vi "Convert Time Stamp to String.vi"(10 "time stamp":timestamp format="%<%Y-%m-%dT%H:%M:%S%8u\nTime zone offset %z>T") -> (3 "date/time string":string)   [LabVIEW 2019, in "infolib.lvlib"]
uses:
  infolib.lvlib
  <vilib>/Utility/miscctls.llb/LVDateTimeRec.ctl
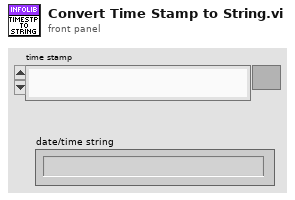
[diagram p1: front panel]
types:
  T1 = typedef "LVDateTimeRec.ctl" = cluster{"fractional second":dbl, "second":i32, "minute":i32, "hour":i32, "day of month":i32, "month":i32, "year":i32, "day of week":i32, "day of year":i32, "DST":i32}
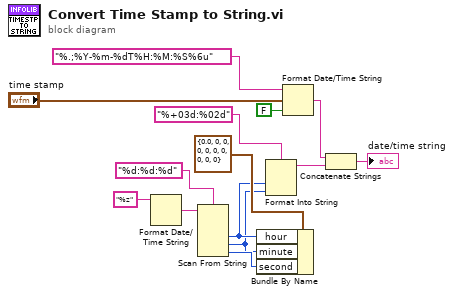
[diagram p0: block diagram]
diagram:
  n1 = Format Date/Time String(time format string (%c)="%z") -> (date/time string=w11:string)  [unwired: 2 in]
  n2 = Scan From String(format string="%d:%d:%d", input string=w11) -> (output 1=w5:i32, output 2=w4:i32, output 3=w8:i32)  [unwired: 5 in, 3 out]
  n3 = Bundle By Name(cluster=T1 {"fractional second"=0.0, "second"=0, "minute"=0, "hour"=0, "day of month"=0, "month"=0, "year"=0, "day of week"=0, "day of year"=0, "DST"=0} ("date time rec"), "hour"=w5, "minute"=w4, "second"=w8) -> ()  [unwired: 1 out]
  n4 = Format Into String(format string="%+03d:%02d", w5, w4) -> (resulting string=w2:string)  [unwired: 2 in, 1 out]
  n5 = Format Date/Time String(time format string (%c)="%.;%Y-%m-%dT%H:%M:%S%6u" ("format string"), seconds (now)="time stamp", UTC format=FALSE) -> (date/time string=w3:string)
  n6 = Concatenate Strings(w3, w2) -> (→"date/time string":string)
